vi "Append Data.vi"(5 "Bit Offset (0)":u32, 6 "Bit Count (0)":u32, 7 "Data Block":string, 8 "error in (no error)":errorcluster, 9 "Destination File":string, 10 "Data Type (0: Generic Data)":i32(ring) items=["Generic Data", "BIT Data"], 11 "VISA resource name":refnum<visa-resource-name>) -> (0 "error out":errorcluster, 3 "VISA resource name out":refnum<visa-resource-name>)   [LabVIEW 2018, in "Agilent PSG MXG Series.lvlib"]
doc: "Append data to an existing file.\n\n<B>Note:</B>\nThis VI is valid on N5171B, N5172B, N5173B, N5181B, N5182B, N5183B, N5161A, N5162A, N5181A, N5182A, N5183A."
uses:
  Agilent PSG MXG Series.lvlib
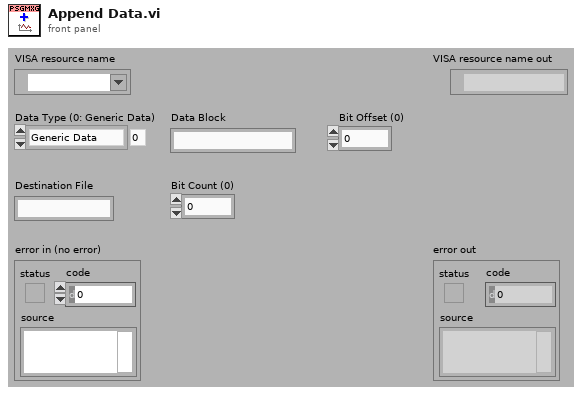
[diagram p1: front panel]
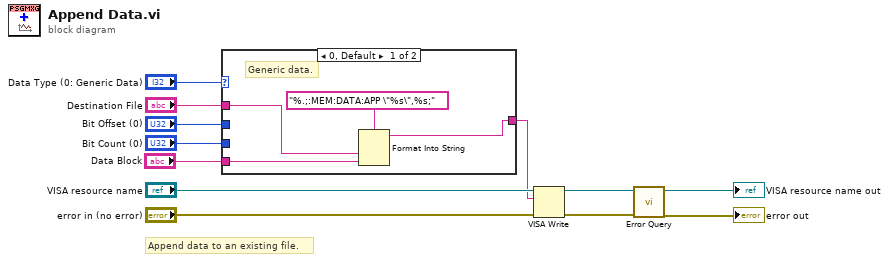
[diagram p0: block diagram]
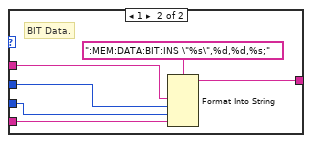
[diagram p2: hidden frame]
diagram:
  # "Append data to an existing file."
  n1 = case shown="0, Default" "Data Type (0: Generic Data)" {
    tunnel: "Destination File" -> [w14 w22]
    tunnel: "Bit Offset (0)" -> [_ w21]
    tunnel: "Bit Count (0)" -> [_ w20]
    tunnel: "Data Block" -> [w13 w19]
    tunnel: [w15 w18] -> w2
    frame 0, Default {
      # "Generic data."
      n2 = Format Into String(format string="%.;:MEM:DATA:APP \"%s\",%s;", w14, w13) -> (resulting string=w15:string)  [unwired: 2 in, 1 out]
    }
    frame 1 {
      # "BIT Data."
      n3 = Format Into String(format string=":MEM:DATA:BIT:INS \"%s\",%d,%d,%s;", w22, w21, w20, w19) -> (resulting string=w18:string)  [unwired: 2 in, 1 out]
    }
  }
  n4 = VISA Write(VISA resource name="VISA resource name", write buffer=w2, error in (no error)="error in (no error)") -> (VISA resource name out=w10:refnum<visa-resource-name>, error out=w9:errorcluster)  [unwired: 1 out]
  n5 = call "Error Query.vi"("error in (no error)"=w9, "VISA resource name"=w10) -> ("error out"=→"error out":errorcluster, "VISA resource name out"=→"VISA resource name out":refnum<visa-resource-name>)  [unwired: 6 in, 2 out]
